vi "Math-Create Rectangle By Center.vi"(0 "x":i16, 7 "y":i16, 11 "size":i16 caption="x") -> (8 "rect":T1)   [LabVIEW 2020]
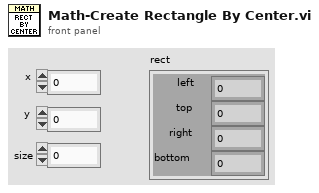
[diagram p1: front panel]
types:
  T1 = cluster{"left":i16, "top":i16, "right":i16, "bottom":i16}
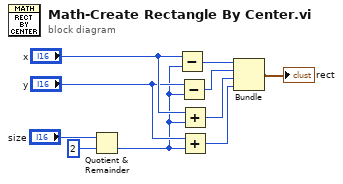
[diagram p0: block diagram]
diagram:
  n1 = Quotient & Remainder(x="size", y=i16 2) -> (floor(x/y)=w1:i16)  [unwired: 1 out]
  n2 = Subtract(x="x", y=w1) -> (x-y=w6:i16)
  n3 = Subtract(x="y", y=w1) -> (x-y=w5:i16)
  n4 = Add(x="x", y=w1) -> (x+y=w4:i16)
  n5 = Add(x="y", y=w1) -> (x+y=w3:i16)
  n6 = Bundle(w6, w5, w4, w3) -> (→"rect":cluster{i16, i16, i16, i16})  [unwired: 1 in]
